vi "模式插入节点.vi"(6 "按键编号":string, 7 "模式input":T1, 8 "动作":string(combo), 9 "按键名字":string(combo), 10 "面板地址":string(combo), 11 "模式选择":string(combo)) -> (3 "模式output":T1)   [LabVIEW 2019]
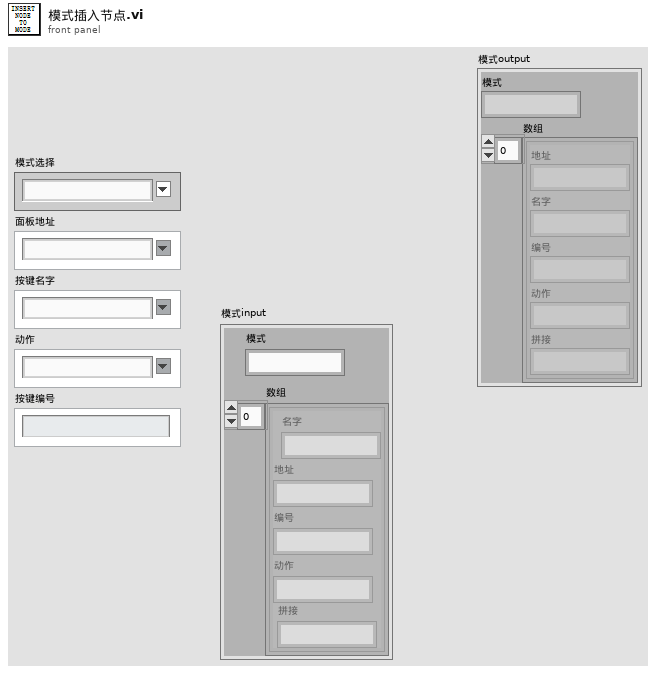
[diagram p1: front panel]
types:
  T1 = cluster{"模式":string, "数组":cluster{"地址":string, "名字":string, "编号":string, "动作":string, "拼接":string}[]}
  T2 = cluster{"地址":string, "名字":string, "编号":string, "动作":string, "拼接":string}[]
  T3 = cluster{"地址":string, "名字":string, "编号":string, "动作":string, "拼接":string}
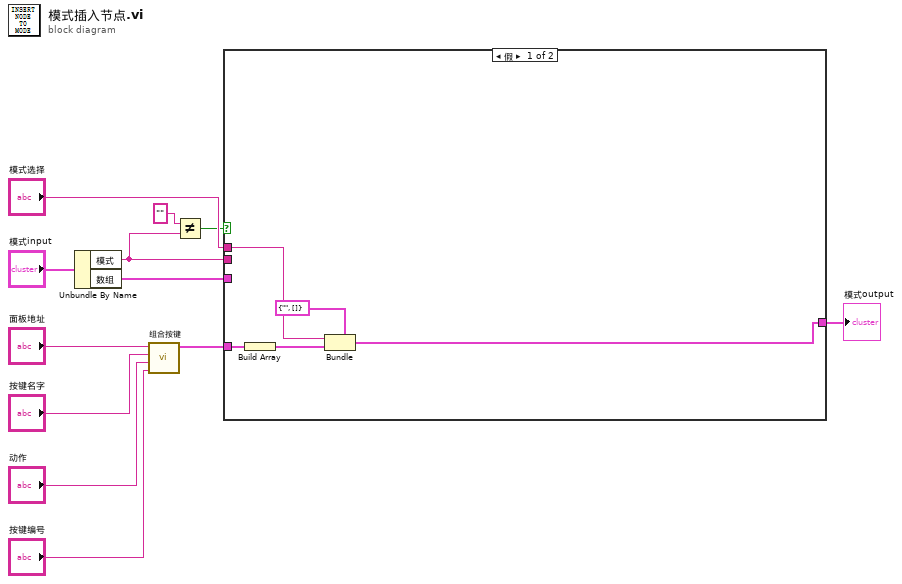
[diagram p0: block diagram]
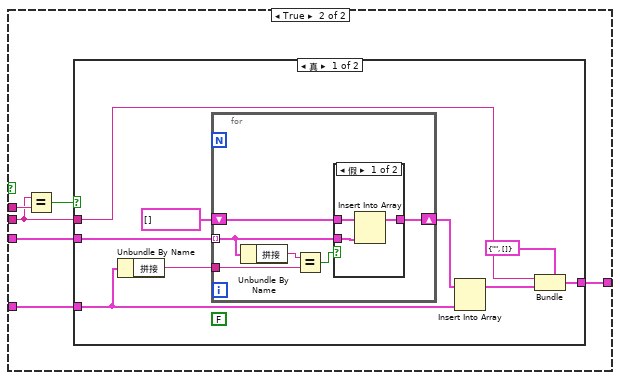
[diagram p2: hidden frame]
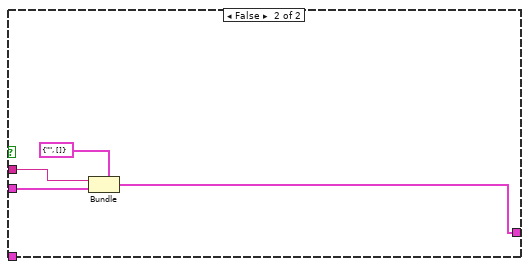
[diagram p4: hidden frame]
diagram:
  n1 = Unbundle By Name("模式input") -> ("模式"=w4:string, "数组"=w6:T2)
  n2 = call "组合按键.vi"("按键编号"="按键编号", "动作"="动作", "按键名字"="按键名字", "面板地址"="面板地址") -> ("按键"=w5:T3)  [unwired: 7 in]
  n3 = Not Equal?(x="", y=w4) -> (x != y?=w1:bool)
  n4 = case shown="假" w1 {
    tunnel: "模式选择" -> [w13 w23]
    tunnel: w6 -> [_ w21]
    tunnel: w5 -> [w17 w20]
    tunnel: w4 -> [_ w19]
    tunnel: [w14 w18] -> w2
    frame False {
      n5 = Build Array(w17) -> (w15:T2)
      n6 = Bundle(cluster=T1 {"模式"="", "数组"=[]} ("模式"), "模式"=w13, "数组"=w15) -> (w14:T1)
    }
    frame True {
      n7 = Equal?(x=w19, y=w23) -> (x = y?=w22:bool)
      n8 = case shown="真" w22 {
        tunnel: w21 -> [w32 w44]
        tunnel: w20 -> [w25 _]
        tunnel: w19 -> [w29 w45]
        tunnel: [w28 w43] -> w18
        frame True {
          (unwired) FALSE
          n9 = Unbundle By Name(w25) -> ("拼接"=w24:string)
          n10 = for {
            tunnel: w32 -> [w34] mode=indexing
            shift-right: [w35] -> w27
            shift-left: T2 [] -> [w36]
            tunnel: w24 -> [w33]
            n11 = Unbundle By Name(w34) -> ("拼接"=w38:string)
            n12 = Equal?(x=w38, y=w33) -> (x = y?=w37:bool)
            n13 = case shown="假" w37 {
              tunnel: w36 -> [w40 w42]
              tunnel: [w41 w42] -> w35
              tunnel: w34 -> [w39 _]
              frame False {
                n14 = Insert Into Array(array=w40, new element=w39) -> (w41:T2)  [unwired: 1 in]
              }
              frame True {
              }
            }
          }
          n15 = Insert Into Array(array=w27, new element=w25) -> (w26:T2)  [unwired: 1 in]
          n16 = Bundle(cluster=T1 {"模式"="", "数组"=[]} ("模式"), "模式"=w29, "数组"=w26) -> (w28:T1)
        }
        frame False {
          n17 = Bundle(cluster=T1 {"模式"="", "数组"=[]} ("模式"), "模式"=w45, "数组"=w44) -> (w43:T1)
        }
      }
    }
  }
  "模式output" <- w2
